vi "Read description.vi"(8 "error in (no error)":errorcluster, 11 "ExampleTask_StopNotifier in":refnum<class "Task_BoolStopNotifier.lvclass">) -> (0 "error out":errorcluster, 2 "description":string, 3 "ExampleTask_StopNotifier out":refnum<class "Task_BoolStopNotifier.lvclass">)   [LabVIEW 2023, in "Task_BoolStopNotifier.lvclass"]
doc: "_____________________________________\nTLC Daemon 1.0.0.2\nCopyright (c) 2026 Andrea Cadei"
uses:
  Task_BoolStopNotifier.lvclass
  Task_BoolStopNotifier.lvclass/Task_BoolStopNotifier.ctl
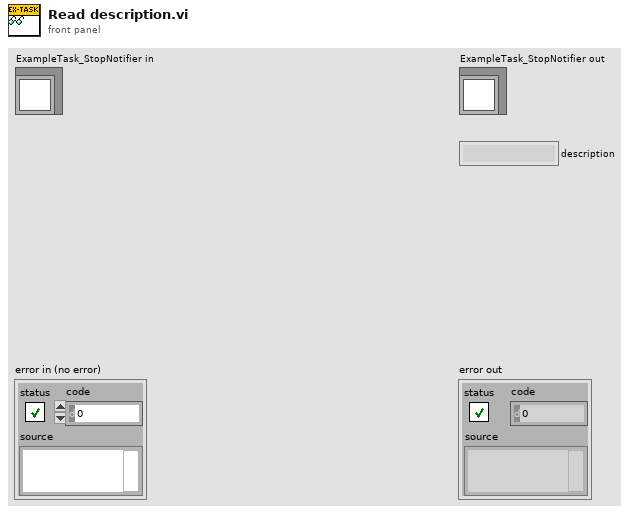
[diagram p1: front panel]
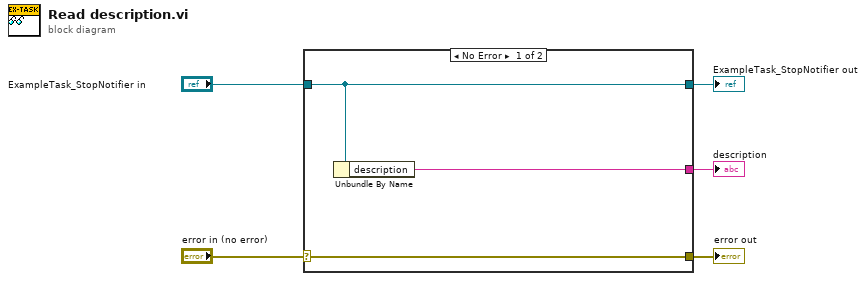
[diagram p0: block diagram]
diagram:
  n1 = case shown="No Error" "error in (no error)" {
    selector: "error in (no error)" -> [w8 w9]
    tunnel: [w8 w9] -> w4
    tunnel: [w7 w10] -> w2
    tunnel: "ExampleTask_StopNotifier in" -> [w7 w10]
    tunnel: [w6 _] -> w1
    frame No Error {
      n2 = Unbundle By Name(w7) -> ("description"=w6:string)
    }
    frame Error {
    }
  }
  "error out" <- w4
  "ExampleTask_StopNotifier out" <- w2
  "description" <- w1
